vi "CAL-Get MAX SPL (click).vi"(5 "Cal path":path, 7 "Sampling Rate (Hz)":dbl, 9 "Npts":i32, 11 "error in (no error)":errorcluster, 12 "Pulse Train Params":T3) -> (8 "Peak SPL":dbl, 15 "error out":errorcluster)   [LabVIEW 2020]
uses:
  epl-vi-lib/Signal Synthesis VIs/Waveform VIs/Pulse Train VIs/Pulse Train Params.ctl
  epl-vi-lib/Signal Synthesis VIs/Waveform VIs/Pulse Train VIs/Pulse Polarity.ctl
  epl-vi-lib/Signal Synthesis VIs/Waveform VIs/Pulse Train VIs/PT-Continuous State.ctl
  epl-vi-lib/Signal Synthesis VIs/Controls/Level XCtl/Level Data.ctl
  epl-vi-lib/Signal Synthesis VIs/Controls/Level XCtl/Level Units.ctl
  epl-vi-lib/Signal Synthesis VIs/Controls/Level XCtl/Level XCtl.xctl
panel:
  in  "Level":T1
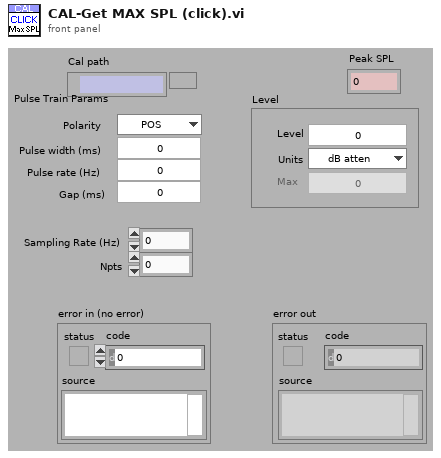
[diagram p1: front panel]
types:
  T1 = typedef "Level XCtl.xctl/Level Data.ctl" = cluster{"Level":dbl, "Units":T2, "Max":dbl, "Multiplier":dbl, "Cal File":path, "Cal":cluster{"Freq (Hz)":dbl[], "Mag (dB SPL)":dbl[], "Phase (deg)":dbl[]}}
  T2 = typedef "Level Units.ctl" = enum16{"dB atten", "dB SPL", "dB re 1 Vrms", "dB V/Hz½", "mW", "dB HL", "Volts", "dB mW"}
  T3 = typedef "Pulse Train Params.ctl" = cluster{"Pulse width (us)":dbl, "Pulse rate (Hz)":dbl, "Gap (ms)":dbl, "Polarity":T4, "PT State":T5, "Asynch":bool}
  T4 = typedef "Pulse Polarity.ctl" = enum16{"POS", "NEG", "POS-NEG", "NEG-POS"}
  T5 = typedef "PT-Continuous State.ctl" = cluster{"Template":dbl[], "Nperiod":i32, "Index":i32, "Pulse Rate (Hz)":dbl, "Phase (cycles)":dbl, "Noff":i32}
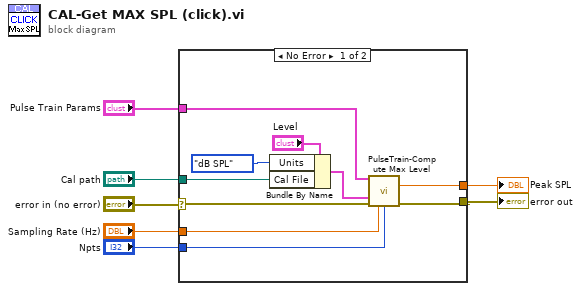
[diagram p0: block diagram]
diagram:
  n1 = case shown="No Error" "error in (no error)" {
    selector: "error in (no error)" -> [w17 w18]
    tunnel: [w11 w18] -> w7
    tunnel: "Pulse Train Params" -> [w16 _]
    tunnel: "Cal path" -> [w14 _]
    tunnel: [w10 _] -> w3
    tunnel: "Sampling Rate (Hz)" -> [w9 _]
    tunnel: "Npts" -> [w8 _]
    frame No Error {
      n2 = Bundle By Name(cluster="Level", "Units"=Level_Units."dB SPL" ("Mode"), "Cal File"=w14) -> (w12:T1)
      n3 = call "PulseTrain-Compute Max Level.vi"("Pulse Train Params"=w16, "Level"=w12, "error in (no error)"=w17, "Sampling Rate (Hz)"=w9, "Npts"=w8) -> ("Max Level"=w10:dbl, "error out"=w11:errorcluster)  [unwired: 8 in, 1 out]
    }
    frame Error {
    }
  }
  "error out" <- w7
  "Peak SPL" <- w3
